vi "Mode enum demo.vi"() -> ()   [LabVIEW 2012]
panel:
  in  "stop":bool
  out "Mode selected":T1(ring)
  in  "Mode":T1(ring)
  # "This is an enum which matches the present state of the Mode select structure \nin \"NXT the tug main C.vI\""
  # "copy this into main code"
  # "Mode 0: motors off, lidar scans from 6-9 (out of 16 positions)\nMode 1: motors on, boat controlled by forebrain arbiter only\nMode 2: motors on, boat controleed by forebrain arbiter and obstacle avoidance\nMode 3:  undesignated. open for use\nMode 4: motors off, set lidar scanning port side\nMode 5: motors on, midbrain doing port wall follow, no forebrain input"
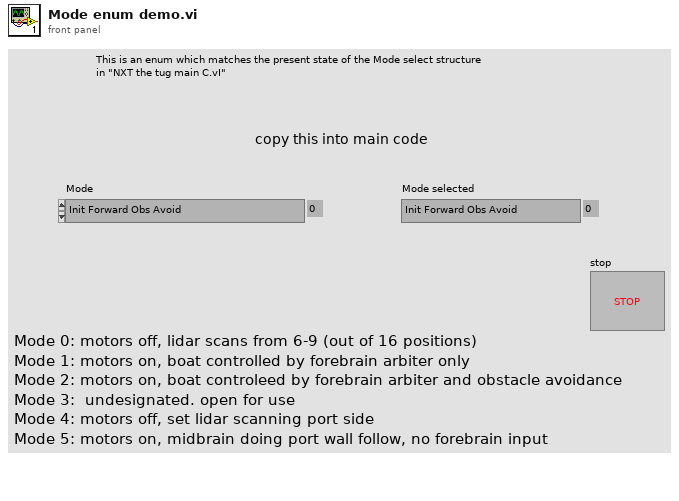
[diagram p1: front panel]
types:
  T1 = enum16{"Init Forward Obs Avoid", "Forebrain Arbiter Only", "FA and FOA", "\"open for use\"", "Init Left H Wall Following", "Left Hand Wall Following"}
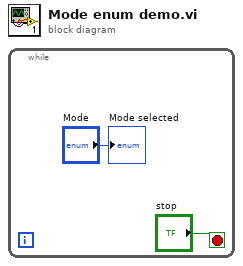
[diagram p0: block diagram]
diagram:
  n1 = while {
    stop <- "stop" stop-if-true
    "Mode selected" <- "Mode"
  }
